vi "ScaledWaveform-AddSection.vi"(8 "Error in":errorcluster, 11 "Custom Device ref":T1 format="%.0x") -> (0 "Error out":errorcluster, 3 "Custom Device ref out":T1 format="%.0x")   [LabVIEW 2020, in "Waveform-Processing-Custom-Device Shared.lvlib" / "Scaled Waveform.lvlib"]
uses:
  Scaled Waveform.lvlib
  <vilib>/NI VeriStand/Custom Device API/Custom Device Item Ref.ctl
  <vilib>/NI VeriStand/Custom Device API/Custom Device Channel.ctl
  <vilib>/NI VeriStand/Custom Device API/Custom Device Channel Type.ctl
  Constants.vi
  <vilib>/NI VeriStand/Custom Device API/Set Item Property (Dependent Node Pointer).vi
  <vilib>/NI VeriStand/Custom Device API/Custom Device API.lvlib
  Waveform-Processing-Custom-Device Shared.lvlib
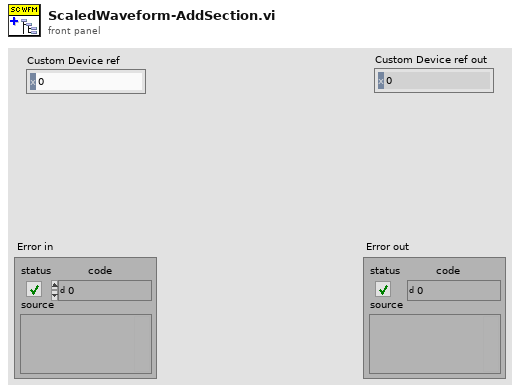
[diagram p1: front panel]
types:
  T1 = typedef "Custom Device API.lvlib/Custom Device Item Ref.ctl" = u64
  T2 = typedef "Custom Device API.lvlib/Custom Device Channel.ctl" = cluster{"Type":T3, "Units":string, "Default Value":dbl, "Faultable":bool, "Scalable":bool}
  T3 = typedef "Custom Device API.lvlib/Custom Device Channel Type.ctl" = enum16{"Input", "Output"}
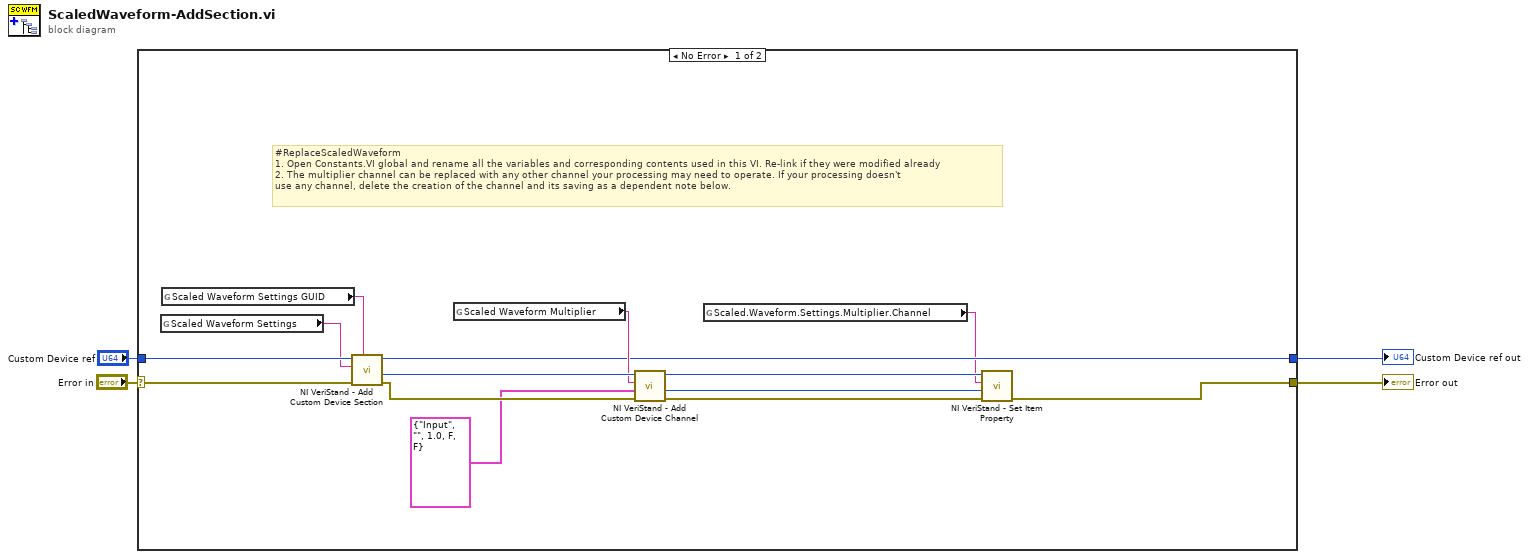
[diagram p0: block diagram]
diagram:
  n1 = case shown="No Error" "Error in" {
    selector: "Error in" -> [w18 w20]
    tunnel: "Custom Device ref" -> [w17 w19]
    tunnel: [w7 w20] -> w2
    tunnel: [w8 w19] -> w1
    frame No Error {
      # "#ReplaceScaledWaveform \n1. Open Constants.VI global and rename all the variables and corresponding contents used in this VI. Re-link if they were modified already \n2. The multiplier channel can be replaced with any other channel your processing may need to operate. If your processing doesn't \nuse any channel, delete the creation of the channel and its saving as a dependent note below."
      n2 = global read "Constants.vi" "Scaled Waveform Settings"() -> (w16:string)
      n3 = global read "Constants.vi" "Scaled Waveform Settings GUID"() -> (w15:string)
      n4 = call <vilib>:"NI VeriStand - Add Custom Device Section.vi"("GUID (Default Section)"=w15, "error in (no error)"=w18, "Section Name"=w16, "Parent Ref in"=w17) -> ("error out"=w13:errorcluster, "Section Ptr"=w14:T1, "Parent Ref out"=w8:T1)  [unwired: 4 in, 1 out]
      n5 = global read "Constants.vi" "Scaled Waveform Multiplier"() -> (w12:string)
      n6 = call <vilib>:"NI VeriStand - Add Custom Device Channel.vi"("error in (no error)"=w13, "Channel"=T2 {"Type"=enum."Input", "Units"="", "Default Value"=1.0, "Faultable"=FALSE, "Scalable"=FALSE}, "Channel Name"=w12, "Parent Ref in"=w14) -> ("error out"=w10:errorcluster, "Channel Ref"=w9:T1, "Parent Ref out"=w11:T1)  [unwired: 4 in, 1 out]
      n7 = global read "Constants.vi" "Scaled.Waveform.Settings.Multiplier.Channel"() -> (w6:string)
      n8 = call-poly <vilib>:"NI VeriStand - Set Item Property.vi"("error in (no error)"=w10, "Dependent Node Ref"=w9, "Property Name"=w6, "Item Ref in"=w11) -> ("error out"=w7:errorcluster)  [unwired: 5 in, 2 out]
    }
    frame Error {
    }
  }
  "Error out" <- w2
  "Custom Device ref out" <- w1
